vi "InterfaceExample.vi"() -> ()   [LabVIEW 2016]
uses:
  <vilib>/rvi/interface/nirviOpenFPGA/nirviOpenFPGA.xnode
  Interface/ScaleAndLimitInterface.lvlib
  Interface/Configuration.ctl
  <vilib>/rvi/interface/nirviReadWriteControl/nirviReadWriteControl.xnode
  <vilib>/rvi/interface/nirviCloseFPGA/nirviCloseFPGA.xnode
  NiFpgaLv.dll
  <vilib>/Utility/error.llb/Error Cluster From Error Code.vi
  <vilib>/rvi/interface/Simulation/niFpgaSimulationCallBeginRW.vi
  <vilib>/rvi/errors/niLvFpgaAdjustHostInterfaceError.vi
  <vilib>/FPGAPlugInAG/Dynamic/niLvFpga_Close_Dynamic.vi
  <instrlib>/_niInstr/FIFO Register Bus/v1/Host/niInstr FIFO Register Bus v1 Host.lvclass
  <instrlib>/_niInstr/Instruction Framework/v1/Host/Subsystem Map/niInstr Subsystem Map v1 Host.lvclass
  C:/Program Files (x86)/National Instruments/LabVIEW 2016/instr.lib/_niInstr/Instruction Framework/v1/Host/Instruction Target/niInstr Instruction Target v1 Host.lvclass
  FPGA Bitfiles/ScaleAndLimit_FPGATarget_BasicExampleWith_-hCiqiYmE3E.lvbitx
  BasicExampleWithInstrFrwk.vi
  <vilib>/FPGAPlugInAG/sbRIO-9607/niLvFpga_Open_sbRIO-9607.vi
  <vilib>/rvi/interface/common/dynamic/niFpgaDynamicAddResources.vi
panel:
  out "ScaledAI":sgl[](array[numeric])
  out "SimultaneousAILoopRate":u32
  in  "DummyChannel15":i16
  in  "stop":bool
  out "Limits":string
  in  "clearLimits":bool
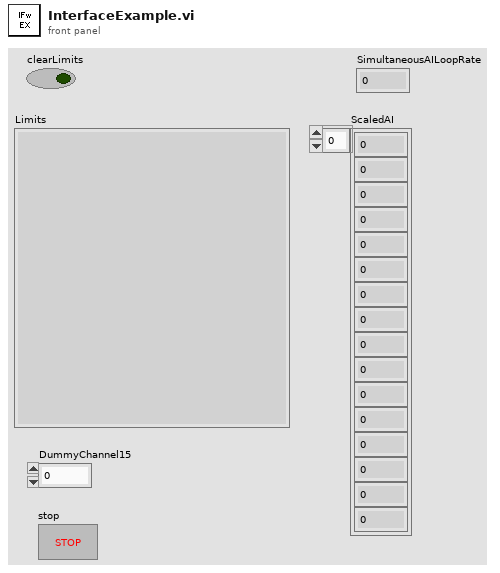
[diagram p1: front panel]
types:
  T1 = typedef "ScaleAndLimitInterface.lvlib/Configuration.ctl" = cluster{"Name":string, "M":dbl, "B":i16, "HighLimit":dbl, "LowLimit":dbl, "LimitsEnabled":bool}
  T2 = typedef "ScaleAndLimitInterface.lvlib/Interface.ctl" = cluster{"instruction target":refnum<class "niInstr Instruction Target v1 Host.lvclass">, "ScalingAndLimitsContext":refnum<class "niInstr Instruction Framework Context v1 Host.lvclass">, "Configuration":T1[]}
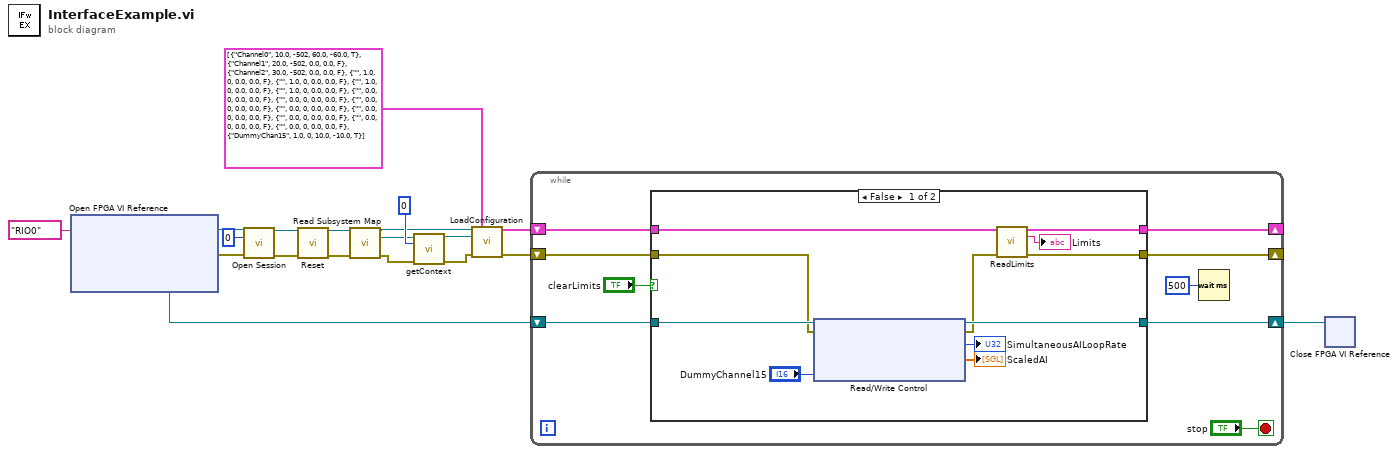
[diagram p0: block diagram]
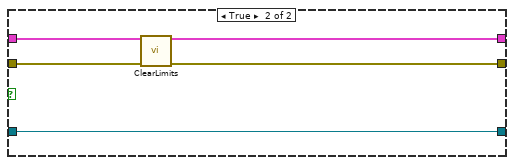
[diagram p2: hidden frame]
diagram:
  n1 = xnode "Open FPGA VI Reference"("resource name"=tag "RIO0") -> ("FPGA VI Reference Out"=w6:refnum<k20>, "error out"=w5:errorcluster)  [unwired: 1 in]
  n2 = call <instrlib>:"Open Session.vi"("fpga ref"=w6, "bus instance"=u32 0, "error in"=w5) -> ("session out"=w9:refnum<class "niInstr FIFO Register Bus v1 Host.lvclass">, "error out"=w10:errorcluster)  [unwired: 11 in]
  n3 = call-dynamic "Reset.vi"("session in"=w9, "error in"=w10) -> ("session out"=w7:refnum<class "niInstr FIFO Register Bus v1 Host.lvclass">, "error out"=w8:errorcluster)  [unwired: 12 in]
  n4 = call <instrlib>:"Read Subsystem Map.vi"("instruction target in"=w7, "error in"=w8) -> ("instruction target out"=w4:refnum<class "niInstr FIFO Register Bus v1 Host.lvclass">, "subsystem map"=w2:refnum<class "niInstr Subsystem Map v1 Host.lvclass">, "error out"=w3:errorcluster)  [unwired: 11 in]
  n5 = call "getContext.vi"("subsystemMap"=w2, "instance"=u8 0, "error in"=w3) -> ("ScalingAndLimitsContext"=w17:refnum<class "niInstr Instruction Framework Context v1 Host.lvclass">, "error out"=w16:errorcluster)  [unwired: 11 in]
  n6 = call "LoadConfiguration.vi"("instruction target in"=w4, "Configuration"=T1[] [{"Name"="Channel0", "M"=10.0, "B"=-502, "HighLimit"=60.0, "LowLimit"=-60.0, "LimitsEnabled"=TRUE}, {"Name"="Channel1", "M"=20.0, "B"=-502, "HighLimit"=0.0, "LowLimit"=0.0, "LimitsEnabled"=FALSE}, {"Name"="Channel2", "M"=30.0, "B"=-502, "HighLimit"=0.0, "LowLimit"=0.0, "LimitsEnabled"=FALSE}, {"Name"="", "M"=1.0, "B"=0, "HighLimit"=0.0, "LowLimit"=0.0, "LimitsEnabled"=FALSE}, {"Name"="", "M"=1.0, "B"=0, "HighLimit"=0.0, "LowLimit"=0.0, "LimitsEnabled"=FALSE}, {"Name"="", "M"=1.0, "B"=0, "HighLimit"=0.0, "LowLimit"=0.0, "LimitsEnabled"=FALSE}, {"Name"="", "M"=1.0, "B"=0, "HighLimit"=0.0, "LowLimit"=0.0, "LimitsEnabled"=FALSE}, {"Name"="", "M"=0.0, "B"=0, "HighLimit"=0.0, "LowLimit"=0.0, "LimitsEnabled"=FALSE}, {"Name"="", "M"=0.0, "B"=0, "HighLimit"=0.0, "LowLimit"=0.0, "LimitsEnabled"=FALSE}, {"Name"="", "M"=0.0, "B"=0, "HighLimit"=0.0, "LowLimit"=0.0, "LimitsEnabled"=FALSE}, {"Name"="", "M"=0.0, "B"=0, "HighLimit"=0.0, "LowLimit"=0.0, "LimitsEnabled"=FALSE}, {"Name"="", "M"=0.0, "B"=0, "HighLimit"=0.0, "LowLimit"=0.0, "LimitsEnabled"=FALSE}, {"Name"="", "M"=0.0, "B"=0, "HighLimit"=0.0, "LowLimit"=0.0, "LimitsEnabled"=FALSE}, {"Name"="", "M"=0.0, "B"=0, "HighLimit"=0.0, "LowLimit"=0.0, "LimitsEnabled"=FALSE}, {"Name"="", "M"=0.0, "B"=0, "HighLimit"=0.0, "LowLimit"=0.0, "LimitsEnabled"=FALSE}, {"Name"="DummyChan15", "M"=1.0, "B"=0, "HighLimit"=10.0, "LowLimit"=-10.0, "LimitsEnabled"=TRUE}], "ScalingAndLimitsContext"=w17, "error in (no error)"=w16) -> ("Interface"=w13:T2, "error out"=w12:errorcluster)  [unwired: 10 in]
  n7 = while {
    shift-right: [w20] -> _
    shift-left: w13 -> [w27]
    shift-right: [w19] -> _
    shift-left: w12 -> [w26]
    shift-right: [w21] -> w11
    shift-left: w6 -> [w22]
    stop <- "stop" stop-if-true
    n8 = case shown="False" "clearLimits" {
      tunnel: w27 -> [w34 w43]
      tunnel: w26 -> [w36 w42]
      tunnel: [w33 w41] -> w20
      tunnel: [w32 w40] -> w19
      tunnel: w22 -> [w38 w39]
      tunnel: [w35 w39] -> w21
      frame False {
        n9 = xnode "Read/Write Control"("FPGA VI Reference In"=w38, "error in"=w36, "DummyChannel15"="DummyChannel15") -> ("FPGA VI Reference Out"=w35:refnum<k20>, "error out"=w30:errorcluster, "SimultaneousAILoopRate"=→"SimultaneousAILoopRate":u32, "ScaledAI"=→"ScaledAI":sgl[])
        n10 = call "ReadLimits.vi"("Interface in"=w34, "error in (no error)"=w30) -> ("Interface out"=w33:T2, "Limits"=→"Limits":string, "error out"=w32:errorcluster)  [unwired: 11 in]
      }
      frame True {
        n11 = call "ClearLimits.vi"("Interface in"=w43, "error in (no error)"=w42) -> ("Interface out"=w41:T2, "error out"=w40:errorcluster)  [unwired: 12 in]
      }
    }
    n12 = Wait (ms)(milliseconds to wait=u32 500) -> ()  [unwired: 1 out]
  }
  n13 = xnode "Close FPGA VI Reference"("FPGA VI Reference In"=w11) -> ()  [unwired: 1 in, 1 out]
